vi "Fit Towel into Design_2.vi"(8 "Towel":T2, 10 "Offset Past Match":i32, 11 "T-Array":T1[](array[typedef])) -> (3 "T-Array Out":T1[](array[typedef]), 5 "Keep Original Out":bool)   [LabVIEW 2024]
uses:
  Cluster_Towel Data_2.ctl
  Cluster_Design Towel ID Data_2.ctl
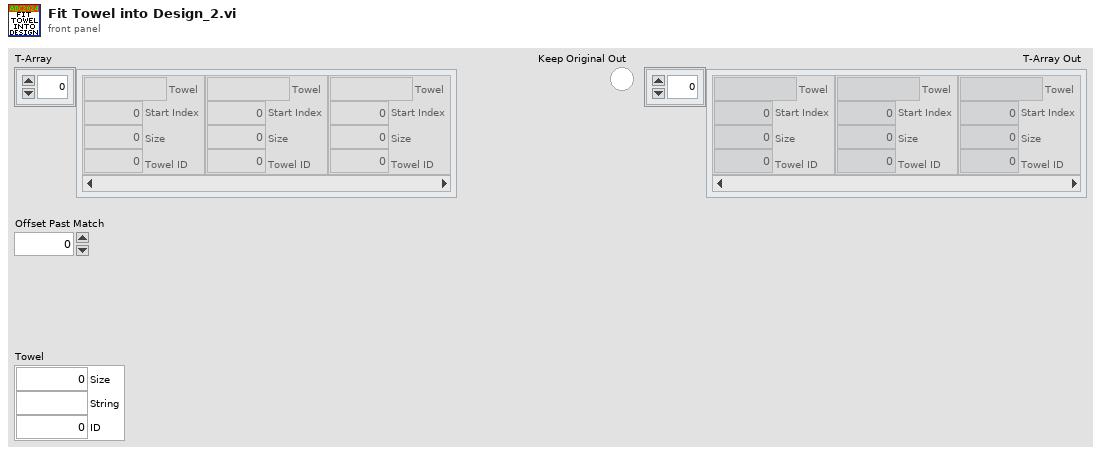
[diagram p1: front panel]
types:
  T1 = typedef "Cluster_Design Towel ID Data_2.ctl" = cluster{"Towel":string, "Start Index":i32, "Size":i32, "Towel ID":i32}
  T2 = typedef "Cluster_Towel Data_2.ctl" = cluster{"Size":i32, "String":string, "ID":i32}
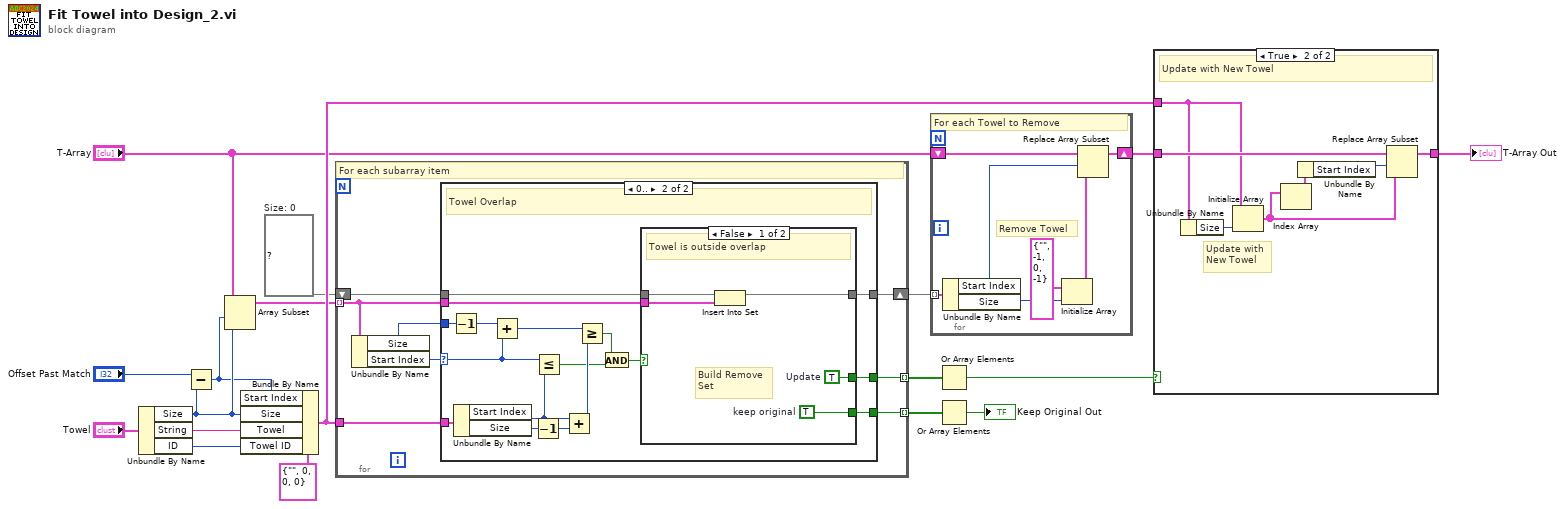
[diagram p0: block diagram]
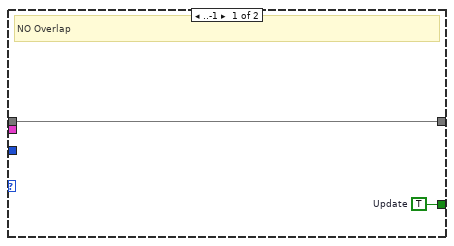
[diagram p3: hidden frame]
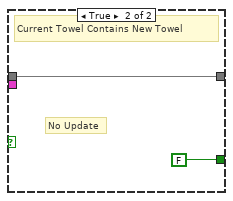
[diagram p4: hidden frame]
diagram:
  w5 = set{T1} {}  # Size: 0
  n1 = Unbundle By Name("Towel") -> ("Size"=w14:i32, "String"=w15:string, "ID"=w17:i32)
  n2 = Subtract(x="Offset Past Match", y=w14) -> (x-y=w11:i32)
  n3 = Array Subset(array="T-Array", index=w11, length=w14) -> (w3:T1[])
  n4 = Bundle By Name(cluster=T1 {"Towel"="", "Start Index"=0, "Size"=0, "Towel ID"=0} ("Tower ID Data"), "Start Index"=w11, "Size"=w14, "Towel"=w15, "Towel ID"=w17) -> (w18:T1)
  n5 = for {
    tunnel: w3 -> [w24] mode=indexing
    tunnel: w18 -> [w20]
    shift-right: [w25] -> w6
    shift-left: w5 -> [w26]
    tunnel: [w21] -> w8 mode=indexing
    tunnel: [w19] -> w2 mode=indexing
    # "For each subarray item"
    n6 = Unbundle By Name(w24) -> ("Size"=w22:i32, "Start Index"=w23:i32)
    n7 = case shown="0.." w23 {
      selector: w23 -> [_ w38]
      tunnel: w26 -> [w28 w45]
      tunnel: [w28 w44] -> w25
      tunnel: w24 -> [_ w43]
      tunnel: w20 -> [_ w42]
      tunnel: w22 -> [_ w39]
      tunnel: [_ w30] -> w21
      tunnel: [w27 w29] -> w19
      frame ..-1 {
        w27 = TRUE  # Update
        # "NO Overlap"
      }
      frame 0.. {
        # "Towel Overlap"
        n8 = Decrement(x=w39) -> (x-1=w37:i32)
        n9 = Unbundle By Name(w42) -> ("Start Index"=w40:i32, "Size"=w41:i32)
        n10 = Add(x=w37, y=w38) -> (x+y=w35:i32)
        n11 = Decrement(x=w41) -> (x-1=w36:i32)
        n12 = Less Or Equal?(x=w38, y=w40) -> (x <= y?=w32:bool)
        n13 = Add(x=w40, y=w36) -> (x+y=w34:i32)
        n14 = Greater Or Equal?(x=w35, y=w34) -> (x >= y?=w33:bool)
        n15 = And(x=w33, y=w32) -> (x .and. y?=w31:bool)
        n16 = case shown="False" w31 {
          tunnel: w45 -> [w50 w52]
          tunnel: [w49 w52] -> w44
          tunnel: w43 -> [w48 _]
          tunnel: [w47 _] -> w30
          tunnel: [w46 FALSE] -> w29
          frame False {
            w46 = TRUE  # Update
            w47 = TRUE  # keep original
            # "Build Remove\nSet"
            # "Towel is outside overlap"
            n17 = Insert Into Set(10:w48, 11:w50) -> (3:w49:set{T1})  [unwired: 1 out]
          }
          frame True {
            # "No Update"
            # "Current Towel Contains New Towel"
          }
        }
      }
    }
  }
  n18 = for {
    tunnel: w6 -> [w58] mode=indexing
    shift-right: [w55] -> w9
    shift-left: "T-Array" -> [w56]
    # "Remove Towel"
    # "For each Towel to Remove"
    n19 = Unbundle By Name(w58) -> ("Start Index"=w54:i32, "Size"=w59:i32)
    n20 = Initialize Array(T1 {"Towel"="", "Start Index"=-1, "Size"=0, "Towel ID"=-1} ("Data"), w59) -> (w53:T1[])
    n21 = Replace Array Subset(array=w56, new element=w53, index=w54) -> (w55:T1[])
  }
  n22 = Or Array Elements(Boolean array=w2) -> (logical OR=w1:bool)
  n23 = Or Array Elements(Boolean array=w8) -> (logical OR=→"Keep Original Out":bool)
  n24 = case shown="True" w1 {
    tunnel: w18 -> [_ w61]
    tunnel: [w60 w63] -> w10
    tunnel: w9 -> [w60 w62]
    frame False {
      # "NO Update"
    }
    frame True {
      # "Update with\nNew Towel"
      # "Update with New Towel"
      n25 = Unbundle By Name(w61) -> ("Size"=w66:i32)
      n26 = Initialize Array(w61, w66) -> (w67:T1[])
      n27 = Index Array(array=w67) -> (element=w64:T1)  [unwired: 1 in]
      n28 = Unbundle By Name(w64) -> ("Start Index"=w65:i32)
      n29 = Replace Array Subset(array=w62, new element=w67, index=w65) -> (w63:T1[])
    }
  }
  "T-Array Out" <- w10
